vi "Main.vi"(11 "Module Admin":refnum<class "Delacor_lib_QMH_Module Admin.lvclass">) -> ()   [LabVIEW 2019, in "CONFIGURATION.lvlib"]
doc: "This template is based off of the Queued Message Handler design pattern and the Queued Message Handler project template that ships with LabVIEW.\n\nThe main difference is that the queue is private to this module and communication between modules is performed via Broadcast and Request events.\n\nRequest events are wrapped in public API methods and are handled in the Event Handling Loop (EHL) of this VI. Any module can register for Broadcast events sent by this module. The EHL generates messages based on user interface actions.\n\nThe Message Handling Loop (MHL) processes messages generated by the EHL, or by other messages. The messages are string values, so new messages can be added easily to the Message Cases case structure in the MHL. Each message cluster can also provide an optional value for Message Data, which is a variant that can be converted to whatever message-specific data is required.\n_____\nBased on Delacor QMH Project Template 5.0.0.82."
uses:
  CONFIGURATION.lvlib
  <vilib>/Delacor/Delacor QMH/Libraries/Module Admin_class/Delacor_lib_QMH_Module Admin.lvclass
  Module Data--cluster.ctl
  Stop Argument--cluster.ctl
  <vilib>/Delacor/Delacor QMH/Libraries/Message Queue_class/Delacor_lib_QMH_Message Queue.lvclass/Delacor_lib_QMH_Message Queue.ctl
  SET CONFIGURATIO Argument--cluster.ctl
  SAVE IN DB Argument--cluster.ctl
  DB_VENDING MACHINE/Type Defs/MONEY.ctl
  DB_VENDING MACHINE/Type Defs/PRODUCTS.ctl
  UPDATE DB TO MONEY LIST Argument--cluster.ctl
  SAVE PRODUCT IN DATABASE Argument--cluster.ctl
  UPDATE DB TO PRODUCT LIST Argument--cluster.ctl
  <vilib>/Utility/miscctls.llb/LVPointTypeDef.ctl
  <vilib>/Delacor/Delacor QMH/Libraries/Module Admin_class/Delacor_lib_QMH_Module Admin.lvclass/Delacor_lib_QMH_Module Admin.ctl
  <vilib>/Delacor/Delacor QMH/Libraries/Message Queue_class/Delacor_lib_QMH_Enqueue Message (Single).vi
  <vilib>/Delacor/Delacor QMH/Libraries/Module Admin_class/Delacor_lib_QMH_Get External Launch.vi
  <vilib>/Utility/error.llb/Error Cluster From Error Code.vi
  <vilib>/ErrorRing/Error Ring.xnode
  <vilib>/Delacor/Delacor QMH/Libraries/Message Queue_class/Delacor_lib_QMH_Message Queue.lvclass
  DB_VENDING MACHINE/DB_VENDING MACHINE.lvlib
  <vilib>/addons/database/NI_Database_API.lvlib
  COINS/COINS.lvlib
  MESSAGES/MESSAGES.lvlib
  Products/Products.lvlib
panel:
  in  "array 2":string[](array[string])
  in  "Tab Control":enum32{"MONEY", "PRODUCTS"}(tab)
  in  "SAVE MONEY IN DATABASE":bool
  in  "REMOVE COIN":bool
  in  "ADD COIN":bool
  in  "VALUE":dbl
  in  "DENOMINATION":string
  in  "Multicolumn MONEY":i32(listbox)
  in  "array":string[](array[string])
  out "MONEY":string[](array[string])
  in  "PRODUCTS":i32(listbox)
  in  "QUANTITY":i8
  in  "COST":dbl
  in  "PRODUCT":string
  in  "DELETE":bool
  in  "SAVE PRODUCT IN DATABASE":bool
  in  "SET CONFIG":bool
  out "error out":errorcluster
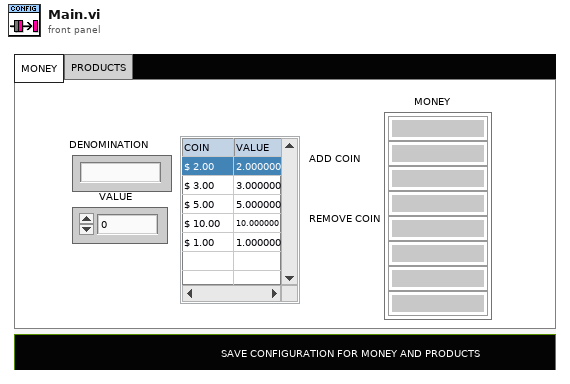
[diagram p1: front panel]
types:
  T1 = typedef "CONFIGURATION.lvlib/Request Events--cluster.ctl" = cluster{"Stop Module":refnum<user-event>, "Show Panel":refnum<user-event>, "Hide Panel":refnum<user-event>, "Get Module Execution Status":refnum<user-event>, "Show Diagram":refnum<user-event>, "SET CONFIGURATIO":refnum<user-event>, "UPDATE DB TO MONEY LIST":refnum<user-event>, "SAVE IN DB":refnum<user-event>, "SAVE PRODUCT IN DATABASE":refnum<user-event>, "UPDATE DB TO PRODUCT LIST":refnum<user-event>}
  T2 = typedef "CONFIGURATION.lvlib/Module Data--cluster.ctl" = cluster{"Status":string, "Money Array":string[]}
  T3 = enum32{"invalid lock state", "Not Locked", "Locked (No Password)", "Password-protected"}
  T4 = typedef "CONFIGURATION.lvlib/Stop Argument--cluster.ctl" = cluster{"Origin":string, "Exit via Stop Module Req?":bool, "Wait for Module to stop?":bool}
  T5 = typedef "CONFIGURATION.lvlib/SET CONFIGURATIO Argument--cluster.ctl" = cluster{"PRODUCTS":cluster{"PRODUCT":string, "COST":dbl, "QUANTITY":i8}, "MONEY":cluster{"COIN":string, "VALUE":dbl}, "MONEY ARRAY":string[]}
  T6 = typedef "DB_VENDING MACHINE.lvlib/MONEY.ctl" = cluster{"COIN":string, "MONEY":dbl}
  T7 = typedef "CONFIGURATION.lvlib/SAVE IN DB Argument--cluster.ctl" = cluster{"MONEY":T6, "PRODUCTS":T8, "DB?":bool}
  T8 = typedef "DB_VENDING MACHINE.lvlib/PRODUCTS.ctl" = cluster{"PRODUCT":string, "COST":dbl, "QUANTITY":i8}
  T9 = typedef "CONFIGURATION.lvlib/UPDATE DB TO MONEY LIST Argument--cluster.ctl" = cluster{"MONEY":T6}
  T10 = typedef "CONFIGURATION.lvlib/SAVE PRODUCT IN DATABASE Argument--cluster.ctl" = cluster{"PRODUCTS":T8}
  T11 = typedef "CONFIGURATION.lvlib/UPDATE DB TO PRODUCT LIST Argument--cluster.ctl" = cluster{"PRODUCTS":T8}
  T12 = enum32{"Invalid", "Standard", "Closed", "Hidden", "Minimized", "Maximized"}
  T13 = cluster{"PRODUCT":string, "COST":dbl, "QUANTITY":i8}
  T14 = typedef "LVPointTypeDef.ctl" = cluster{"Horizontal":i16, "Vertical":i16}
  T15 = typedef "NI_Database_API.lvlib/Conn ObjectReference.ctl" = refnum<k1>
  T16 = cluster{"array 2[0]":string, "array 2[1]":string, "array 2[2]":string, "array 2[3]":string, "array 2[4]":string, "array 2[5]":string, "array 2[6]":string, "array 2[7]":string, "array 2[8]":string}
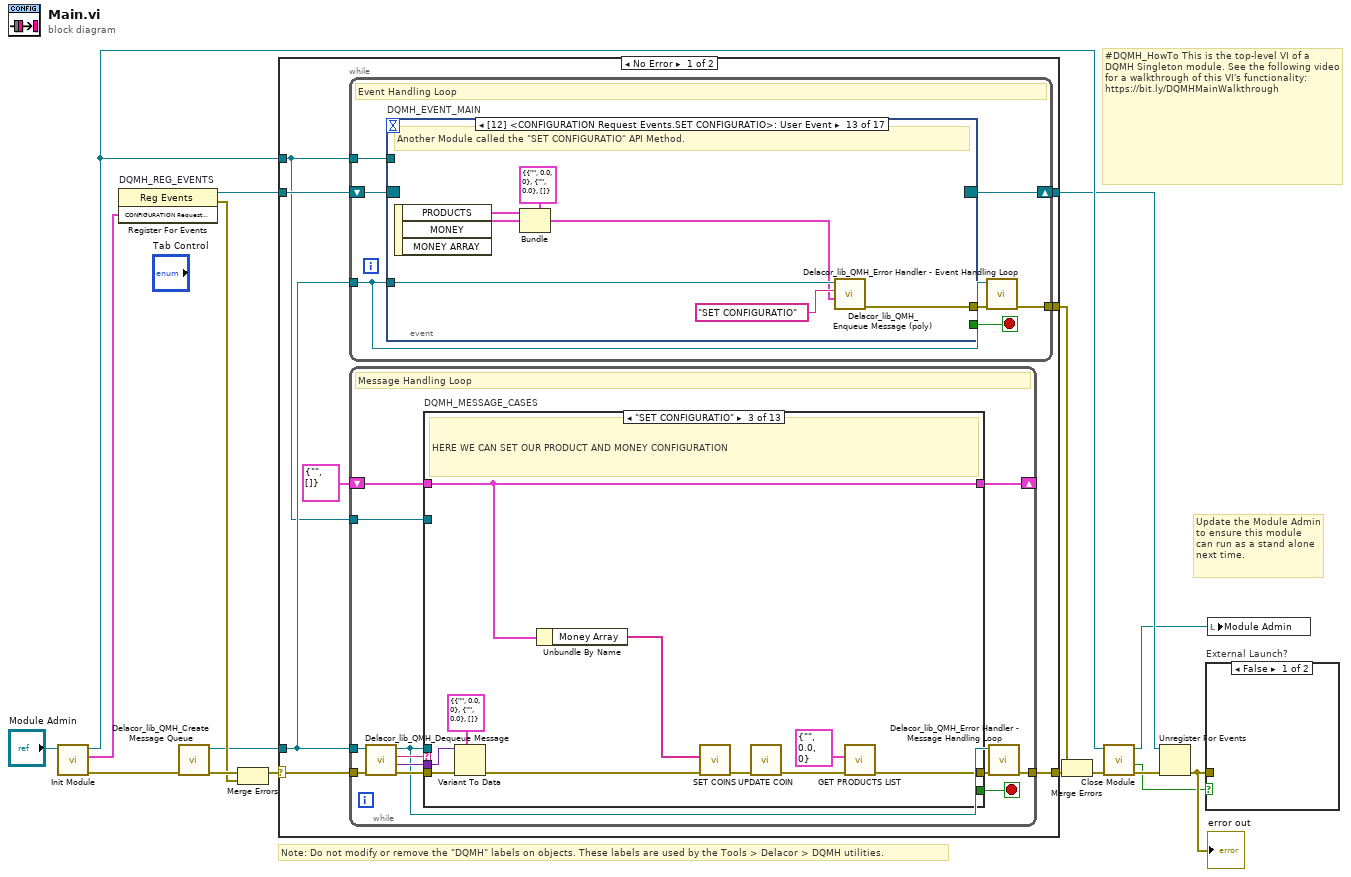
[diagram p0: block diagram]
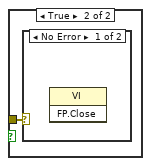
[diagram p2: hidden frame]
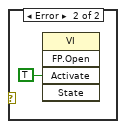
[diagram p3: hidden frame]
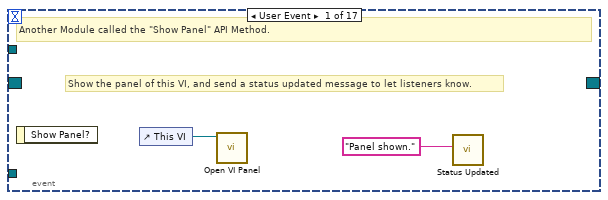
[diagram p4: hidden frame]
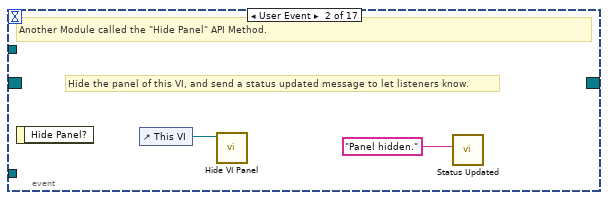
[diagram p5: hidden frame]
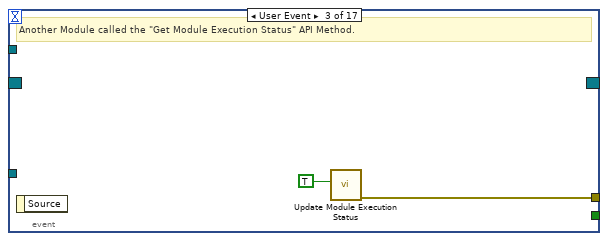
[diagram p6: hidden frame]
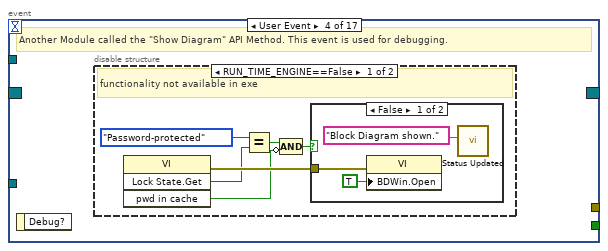
[diagram p7: hidden frame]
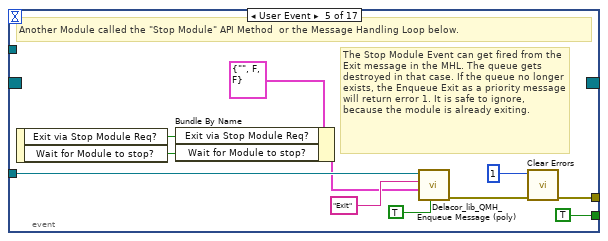
[diagram p10: hidden frame]
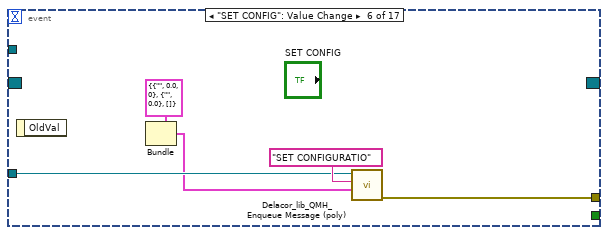
[diagram p11: hidden frame]
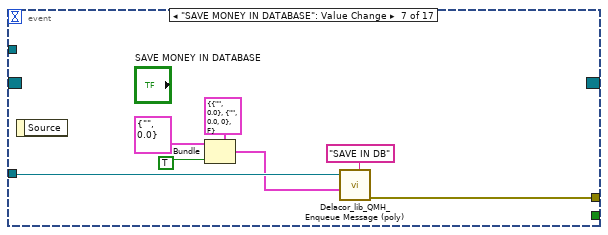
[diagram p12: hidden frame]
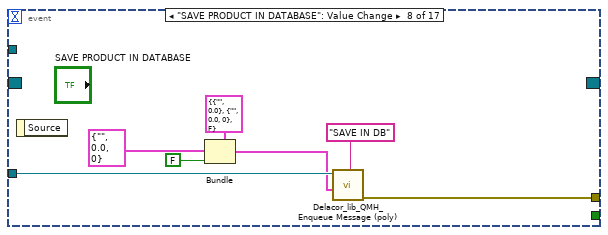
[diagram p13: hidden frame]
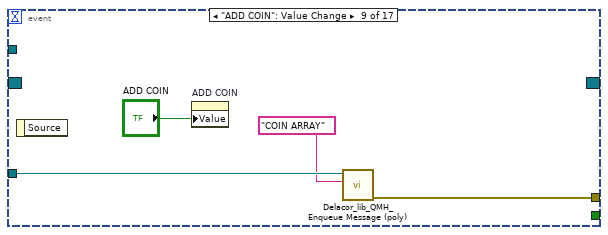
[diagram p14: hidden frame]
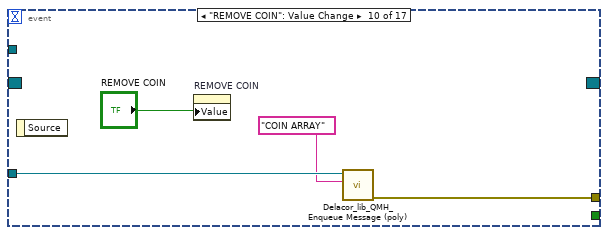
[diagram p15: hidden frame]
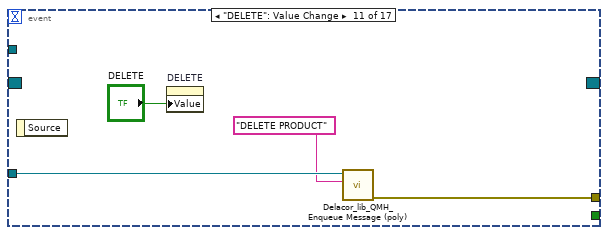
[diagram p16: hidden frame]
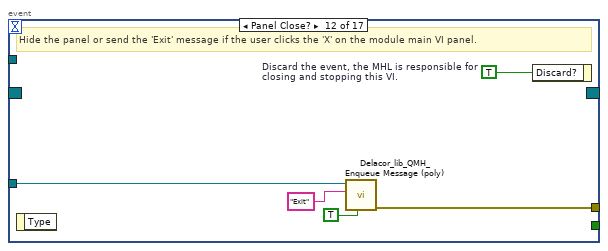
[diagram p17: hidden frame]
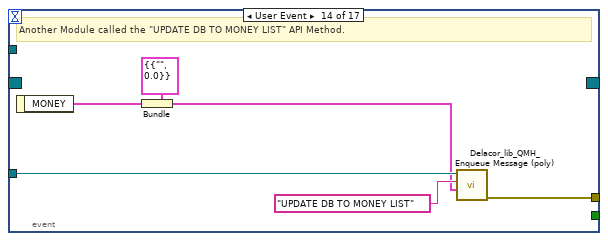
[diagram p18: hidden frame]
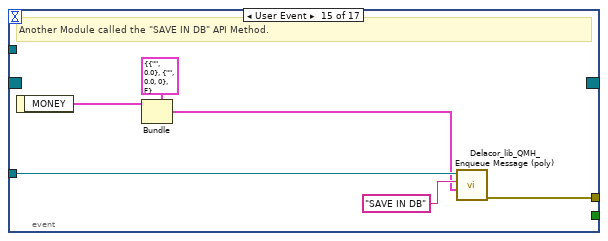
[diagram p19: hidden frame]
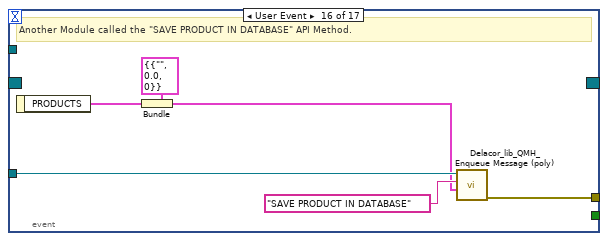
[diagram p20: hidden frame]
diagram:
  # "#DQMH_HowTo This is the top-level VI of a DQMH Singleton module. See the following video for a walkthrough of this VI's functionality: https://bit.ly/DQMHMainWalkthrough"
  # "Note: Do not modify or remove the \"DQMH\" labels on objects. These labels are used by the Tools > Delacor > DQMH utilities."
  # "Update the Module Admin to ensure this module can run as a stand alone next time."
  n1 = call "Init Module.vi"("Singleton Module Admin in"="Module Admin") -> ("error out"=w16:errorcluster, "CONFIGURATION Request Events"=w5:T1, "Singleton Module Admin out"=w8:refnum<class "Delacor_lib_QMH_Module Admin.lvclass">)  [unwired: 8 in]
  n2 = register-events "DQMH_REG_EVENTS"(w5) -> (reference out=w6:refnum<event-registration>, error out=w9:errorcluster)  [unwired: 2 in]
  n3 = call <vilib>:"Delacor_lib_QMH_Create Message Queue.vi"("error in (no error)"=w16) -> ("error out"=w11:errorcluster, "Message Queue"=w4:refnum<class "Delacor_lib_QMH_Message Queue.lvclass">)  [unwired: 9 in]
  n4 = Merge Errors(w11, w9) -> (w10:errorcluster)
  n5 = case shown="No Error" w10 {
    selector: w10 -> [w23 w320]
    tunnel: [w25 w319] -> w17
    tunnel: [w22 w325] -> w7
    tunnel: w6 -> [w20 w325]
    tunnel: w4 -> [w19 w318]
    tunnel: [w24 _] -> w14
    tunnel: w8 -> [w18 w321]
    frame No Error {
      n6 = while {
        tunnel: w19 -> [w26]
        shift-right: [w29] -> w22
        shift-left: w20 -> [w30]
        tunnel: [w31] -> w24
        tunnel: w18 -> [w27]
        stop <- w28 stop-if-true
        # "Event Handling Loop"
        n7 = event "DQMH_EVENT_MAIN" shown="[12] <CONFIGURATION Request Events.SET CONFIGURATIO>: User Event" {
          selector: w30 -> [_ _ _ _ _ _ _ _ _ _ _ _ _ _ _ _ _]
          dyn-events: [_ _ _ _ _ _ _ _ _ _ _ _ _ _ _ _ _] -> w29
          timeout: _ -> [_ _ _ _ _ _ _ _ _ _ _ _ _ _ _ _ _]
          tunnel: [_ _ _ _ TRUE ("Discard?") _ _ _ _ _ _ _ _ _ _ _ _] -> w28
          tunnel: w26 -> [_ _ _ _ w54 w62 w66 w72 w81 w85 w89 w92 w101 w107 w113 w119 w125]
          tunnel: [_ _ w38 _ w57 w61 w64 w73 w78 w82 w86 w94 w95 w102 w108 w114 w120] -> w32
          tunnel: w27 -> [_ _ _ _ _ _ _ _ _ _ _ _ _ _ _ _ _]
          event User Event {
            # "Show the panel of this VI, and send a status updated message to let listeners know."
            # "Another Module called the \"Show Panel\" API Method."
            n8 = event-data() -> ()  [unwired: 1 in, 1 out]
            n9 = control-ref of="This VI"() -> (w34:refnum<vi>)
            n10 = call "Open VI Panel.vi"("VI"=w34) -> ()  [unwired: 10 in, 1 out]
            n11 = call "Status Updated.vi"("Status"="Panel shown." ("format string")) -> ()  [unwired: 10 in, 1 out]
          }
          event User Event {
            # "Hide the panel of this VI, and send a status updated message to let listeners know."
            # "Another Module called the \"Hide Panel\" API Method."
            n12 = event-data() -> ()  [unwired: 1 in, 1 out]
            n13 = control-ref of="This VI"() -> (w36:refnum<vi>)
            n14 = call "Hide VI Panel.vi"("VI"=w36) -> ()  [unwired: 10 in, 1 out]
            n15 = call "Status Updated.vi"("Status"="Panel hidden." ("format string")) -> ()  [unwired: 10 in, 1 out]
          }
          event User Event {
            # "Another Module called the \"Get Module Execution Status\" API Method."
            n16 = event-data() -> ()  [unwired: 1 in, 1 out]
            n17 = call "Update Module Execution Status.vi"("Running?"=TRUE) -> ("error out"=w38:errorcluster)  [unwired: 10 in]
          }
          event User Event {
            # "Another Module called the \"Show Diagram\" API Method. This event is used for debugging."
            n18 = event-data() -> ()  [unwired: 1 in, 1 out]
            n19 = disable-structure shown="RUN_TIME_ENGINE==False" {
              frame condition #0 (active) {
                # "functionality not available in exe"
                n20 = invoke class="VI" method="Lock State.Get"() -> (error out=w44:errorcluster, "Get Lock State"=w43:T3, "pwd in cache"=w40:bool)  [unwired: 4 in, 1 out]
                n21 = Equal?(x=T3."Password-protected", y=w43) -> (x = y?=w41:bool)
                n22 = Compound Arithmetic op=AND(w41, invert w40) -> (w39:bool)
                n23 = case shown="False" w39 {
                  tunnel: w44 -> [w47 _]
                  frame False {
                    n24 = property class="VI"(error in=w47, "BDWin.Open"=TRUE ("Block Diagram Window:Open")) -> ()  [unwired: 1 in, 2 out]
                    n25 = call "Status Updated.vi"("Status"="Block Diagram shown." ("format string")) -> ()  [unwired: 10 in, 1 out]
                  }
                  frame True {
                    # "Password-protected VI, and the password is not in the cache. Do not show the diagram."
                  }
                }
              }
              frame condition #1 {
              }
            }
          }
          event User Event {
            # "The Stop Module Event can get fired from the Exit message in the MHL. The queue gets destroyed in that case. If the queue no longer exists, the Enqueue Exit as a priority message will return error 1. It is safe to ignore, because the module is already exiting."
            # "Another Module called the \"Stop Module\" API Method  or the Message Handling Loop below."
            n26 = event-data() -> ("Exit via Stop Module Req?"=w50:bool, "Wait for Module to stop?"=w49:bool)  [unwired: 1 in]
            n27 = Bundle By Name(cluster=T4 {"Origin"="", "Exit via Stop Module Req?"=FALSE, "Wait for Module to stop?"=FALSE} ("Stop Argument"), "Exit via Stop Module Req?"=w50, "Wait for Module to stop?"=w49) -> (w48:T4)
            n28 = call-poly <vilib>:"Delacor_lib_QMH_Enqueue Message (poly).vi"("Priority Message? (F)"=TRUE, "Message Data"=w48, "Message"="Exit", "Message Queue in"=w54) -> ("error out"=w58:errorcluster)  [unwired: 6 in, 1 out]
            n29 = call <vilib>:"Clear Errors.vi"("error in (no error)"=w58, "specific error code to clear (0: all)"=1) -> ("error out"=w57:errorcluster)  [unwired: 4 in, 1 out]
          }
          event "SET CONFIG": Value Change {
            n30 = event-data() -> ()  [unwired: 1 in, 1 out]
            n31 = Bundle(cluster=T5 {"PRODUCTS"={"PRODUCT"="", "COST"=0.0, "QUANTITY"=0}, "MONEY"={"COIN"="", "VALUE"=0.0}, "MONEY ARRAY"=[]} ("SET CONFIGURATIO Argument")) -> (w59:T5)  [unwired: 3 in]
            n32 = call-poly <vilib>:"Delacor_lib_QMH_Enqueue Message (poly).vi"("Message Data"=w59, "Message"="SET CONFIGURATIO", "Message Queue in"=w62) -> ("error out"=w61:errorcluster)  [unwired: 7 in, 1 out]
          }
          event "SAVE MONEY IN DATABASE": Value Change {
            n33 = event-data() -> ()  [unwired: 1 in, 1 out]
            n34 = Bundle(cluster=T7 {"MONEY"={"COIN"="", "MONEY"=0.0}, "PRODUCTS"={"PRODUCT"="", "COST"=0.0, "QUANTITY"=0}, "DB?"=FALSE} ("SAVE IN DB Argument"), "MONEY"=T6 {"COIN"="", "MONEY"=0.0}, "DB?"=TRUE) -> (w65:T7)  [unwired: 1 in]
            n35 = call-poly <vilib>:"Delacor_lib_QMH_Enqueue Message (poly).vi"("Message Data"=w65, "Message"="SAVE IN DB", "Message Queue in"=w66) -> ("error out"=w64:errorcluster)  [unwired: 7 in, 1 out]
          }
          event "SAVE PRODUCT IN DATABASE": Value Change {
            n36 = event-data() -> ()  [unwired: 1 in, 1 out]
            n37 = Bundle(cluster=T7 {"MONEY"={"COIN"="", "MONEY"=0.0}, "PRODUCTS"={"PRODUCT"="", "COST"=0.0, "QUANTITY"=0}, "DB?"=FALSE} ("SAVE IN DB Argument"), "PRODUCTS"=T8 {"PRODUCT"="", "COST"=0.0, "QUANTITY"=0}, "DB?"=FALSE) -> (w71:T7)  [unwired: 1 in]
            n38 = call-poly <vilib>:"Delacor_lib_QMH_Enqueue Message (poly).vi"("Message Data"=w71, "Message"="SAVE IN DB", "Message Queue in"=w72) -> ("error out"=w73:errorcluster)  [unwired: 7 in, 1 out]
          }
          event "ADD COIN": Value Change {
            n39 = event-data() -> ()  [unwired: 1 in, 1 out]
            n40 = property on="ADD COIN" class="Bool (strict)"("Value"="ADD COIN") -> ()  [unwired: 2 in, 2 out]
            n41 = call-poly <vilib>:"Delacor_lib_QMH_Enqueue Message (poly).vi"("Message"="COIN ARRAY", "Message Queue in"=w81) -> ("error out"=w78:errorcluster)  [unwired: 8 in, 1 out]
          }
          event "REMOVE COIN": Value Change {
            n42 = event-data() -> ()  [unwired: 1 in, 1 out]
            n43 = property on="REMOVE COIN" class="Bool (strict)"("Value"="REMOVE COIN") -> ()  [unwired: 2 in, 2 out]
            n44 = call-poly <vilib>:"Delacor_lib_QMH_Enqueue Message (poly).vi"("Message"="COIN ARRAY", "Message Queue in"=w85) -> ("error out"=w82:errorcluster)  [unwired: 8 in, 1 out]
          }
          event "DELETE": Value Change {
            n45 = event-data() -> ()  [unwired: 1 in, 1 out]
            n46 = property on="DELETE" class="Bool (strict)"("Value"="DELETE") -> ()  [unwired: 2 in, 2 out]
            n47 = call-poly <vilib>:"Delacor_lib_QMH_Enqueue Message (poly).vi"("Message"="DELETE PRODUCT", "Message Queue in"=w89) -> ("error out"=w86:errorcluster)  [unwired: 8 in, 1 out]
          }
          event Panel Close? {
            w93 = TRUE  # Discard the event, the MHL is responsible for closing and stopping this VI.
            # "Hide the panel or send the 'Exit' message if the user clicks the 'X' on the module main VI panel."
            n48 = event-data() -> ()  [unwired: 1 in, 1 out]
            n49 = call-poly <vilib>:"Delacor_lib_QMH_Enqueue Message (poly).vi"("Priority Message? (F)"=TRUE, "Message"="Exit", "Message Queue in"=w92) -> ("error out"=w94:errorcluster)  [unwired: 7 in, 1 out]
            n50 = event-data("Discard?"=w93) -> ()  [unwired: 1 in, 1 out]
          }
          event User Event {
            # "Another Module called the \"SET CONFIGURATIO\" API Method."
            n51 = event-data() -> ("PRODUCTS"=w97:T13, "MONEY"=w96:cluster{"COIN":string, "VALUE":dbl})  [unwired: 1 in, 1 out]
            n52 = Bundle(cluster=T5 {"PRODUCTS"={"PRODUCT"="", "COST"=0.0, "QUANTITY"=0}, "MONEY"={"COIN"="", "VALUE"=0.0}, "MONEY ARRAY"=[]} ("SET CONFIGURATIO Argument"), "PRODUCTS"=w97, "MONEY"=w96) -> (w98:T5)  [unwired: 1 in]
            n53 = call-poly <vilib>:"Delacor_lib_QMH_Enqueue Message (poly).vi"("Message Data"=w98, "Message"="SET CONFIGURATIO", "Message Queue in"=w101) -> ("error out"=w95:errorcluster)  [unwired: 7 in, 1 out]
          }
          event User Event {
            # "Another Module called the \"UPDATE DB TO MONEY LIST\" API Method."
            n54 = event-data() -> ("MONEY"=w103:T6)  [unwired: 1 in]
            n55 = Bundle(cluster=T9 {"MONEY"={"COIN"="", "MONEY"=0.0}} ("UPDATE DB TO MONEY LIST Argument"), "MONEY"=w103) -> (w104:T9)
            n56 = call-poly <vilib>:"Delacor_lib_QMH_Enqueue Message (poly).vi"("Message Data"=w104, "Message"="UPDATE DB TO MONEY LIST", "Message Queue in"=w107) -> ("error out"=w102:errorcluster)  [unwired: 7 in, 1 out]
          }
          event User Event {
            # "Another Module called the \"SAVE IN DB\" API Method."
            n57 = event-data() -> ("MONEY"=w109:T6)  [unwired: 1 in]
            n58 = Bundle(cluster=T7 {"MONEY"={"COIN"="", "MONEY"=0.0}, "PRODUCTS"={"PRODUCT"="", "COST"=0.0, "QUANTITY"=0}, "DB?"=FALSE} ("SAVE IN DB Argument"), "MONEY"=w109) -> (w110:T7)  [unwired: 2 in]
            n59 = call-poly <vilib>:"Delacor_lib_QMH_Enqueue Message (poly).vi"("Message Data"=w110, "Message"="SAVE IN DB", "Message Queue in"=w113) -> ("error out"=w108:errorcluster)  [unwired: 7 in, 1 out]
          }
          event User Event {
            # "Another Module called the \"SAVE PRODUCT IN DATABASE\" API Method."
            n60 = event-data() -> ("PRODUCTS"=w115:T8)  [unwired: 1 in]
            n61 = Bundle(cluster=T10 {"PRODUCTS"={"PRODUCT"="", "COST"=0.0, "QUANTITY"=0}} ("SAVE PRODUCT IN DATABASE Argument"), "PRODUCTS"=w115) -> (w116:T10)
            n62 = call-poly <vilib>:"Delacor_lib_QMH_Enqueue Message (poly).vi"("Message Data"=w116, "Message"="SAVE PRODUCT IN DATABASE", "Message Queue in"=w119) -> ("error out"=w114:errorcluster)  [unwired: 7 in, 1 out]
          }
          event User Event {
            # "Another Module called the \"UPDATE DB TO PRODUCT LIST\" API Method."
            n63 = event-data() -> ("PRODUCTS"=w121:T8)  [unwired: 1 in]
            n64 = Bundle(cluster=T11 {"PRODUCTS"={"PRODUCT"="", "COST"=0.0, "QUANTITY"=0}} ("UPDATE DB TO PRODUCT LIST Argument"), "PRODUCTS"=w121) -> (w122:T11)
            n65 = call-poly <vilib>:"Delacor_lib_QMH_Enqueue Message (poly).vi"("Message Data"=w122, "Message"="UPDATE DB TO PRODUCT LIST", "Message Queue in"=w125) -> ("error out"=w120:errorcluster)  [unwired: 7 in, 1 out]
          }
        }
        n66 = call-dynamic "Delacor_lib_QMH_Error Handler - Event Handling Loop.vi"("error in (no error)"=w32, "Message Queue in"=w26) -> ("dup error in"=w31:errorcluster)  [unwired: 8 in, 1 out]
      }
      n67 = while {
        tunnel: w19 -> [w128]
        shift-right: [w132] -> _
        shift-left: T2 {"Status"="", "Money Array"=[]} ("Data Cluster") -> [w133]
        tunnel: w23 -> [w136]
        tunnel: [w134] -> w25
        tunnel: w18 -> [w126]
        stop <- w131 stop-if-true
        # "Message Handling Loop"
        n68 = call-dynamic "Delacor_lib_QMH_Dequeue Message.vi"("error in (no error)"=w136, "Message Queue in"=w128) -> ("error out"=w135:errorcluster, "Message Data"=w129:variant, "Message"=w130:string, "Message Queue out"=w127:refnum<class "Delacor_lib_QMH_Message Queue.lvclass">)  [unwired: 6 in]
        n69 = case "DQMH_MESSAGE_CASES" shown="\"SET CONFIGURATIO\"" w130 {
          selector: w130 -> [_ _ _ _ _ _ _ _ _ _ _ _ w305]
          tunnel: w127 -> [_ _ _ _ _ _ _ _ _ _ w275 w297 _]
          tunnel: w135 -> [w157 w161 w171 w185 w197 w214 w242 w266 w269 w271 w282 w303 w307]
          tunnel: [w140 w161 w163 w174 w186 w214 w241 w255 w268 w271 w278 w300 w308] -> w137
          tunnel: w133 -> [w147 w160 w168 w184 w196 w217 w243 w253 w267 w270 w277 w296 w306]
          tunnel: [w147 w160 w168 w184 w196 w216 w243 w253 w267 w270 w277 w296 w306] -> w132
          tunnel: [_ _ _ _ _ _ _ _ _ _ _ w295 _] -> w131
          tunnel: w129 -> [_ _ w170 w182 w195 _ _ w264 _ _ w276 w294 _]
          tunnel: w126 -> [w148 _ _ _ _ _ _ _ _ _ w274 w289 _]
          frame "Initialize" {
            (unwired) T14 {"Horizontal"=0, "Vertical"=0} ("Origin")
            # "Initialize - Any operation that needs to be done before the module can receive messages. Synchronize Caller Events.vi will inform Start Module.vi that the module has launched and is ready to receive messages. Module Did Init.vi will broadcast that the module initialized."
            n70 = call "Synchronize Caller Events.vi"("error in (no error)"=w157, "Singleton Module Admin in"=w148) -> ("error out"=w156:errorcluster, "Singleton Module Admin out"=w144:refnum<class "Delacor_lib_QMH_Module Admin.lvclass">)  [unwired: 8 in]
            n71 = property class="Module Admin"(reference=w144) -> ("Accessors:External Launch"=w152:bool)  [unwired: 1 in, 2 out]
            n72 = Select(t=T12."Hidden" ("State"), s=w152, f=T12."Standard" ("State")) -> (s? t:f=w149:T12)
            n73 = call "Module Name--constant.vi"() -> ("Module Name"=w145:string)  [unwired: 11 in]
            n74 = call "SET MESSAGE.vi"("Message"="SETTING UP VENDING MACHINE") -> ()  [unwired: 10 in, 1 out]
            n75 = call "Module Name--constant.vi"() -> ("Module Name"=w155:string)  [unwired: 11 in]
            n76 = call "Module Did Init.vi"("error in (no error)"=w156, "Initialized?"=TRUE, "Origin"=w145) -> ("error out"=w143:errorcluster)  [unwired: 8 in]
            n77 = property class="VI"("Front Panel.Title"=w155) -> (reference out=w154:refnum<vi>, error out=w159:errorcluster)  [unwired: 2 in]
            n78 = invoke class="VI" method="FP.Open"(reference=w154, error in=w159, "State"=w149) -> (reference out=w153:refnum<vi>, error out=w158:errorcluster)  [unwired: 2 in, 3 out]
            n79 = call "UPDATE DB TO MONEY LIST.vi"("error in (no error)"=w143, "MONEY"=T6 {"COIN"="", "MONEY"=0.0}) -> ("error out"=w142:errorcluster)  [unwired: 9 in]
            n80 = invoke class="VI" method="FP.Center"(reference=w153, error in=w158) -> ()  [unwired: 1 in, 3 out]
            n81 = call "UPDATE DB TO PRODUCT LIST.vi"("error in (no error)"=w142, "PRODUCTS"=T8 {"PRODUCT"="", "COST"=0.0, "QUANTITY"=0}) -> ("error out"=w140:errorcluster)  [unwired: 9 in]
          }
          frame "--- Module Specific ---" {
            # "Separator -- The following cases handle messages specific to this Module."
          }
          frame "SET CONFIGURATIO" {
            # "HERE WE CAN SET OUR PRODUCT AND MONEY CONFIGURATION"
            n82 = Variant To Data(error in=w171, type=T5 {"PRODUCTS"={"PRODUCT"="", "COST"=0.0, "QUANTITY"=0}, "MONEY"={"COIN"="", "VALUE"=0.0}, "MONEY ARRAY"=[]} ("SET CONFIGURATIO Argument"), Variant=w170) -> (error out=w165:errorcluster)  [unwired: 1 out]
            n83 = Unbundle By Name(w168) -> ("Money Array"=w167:string[])
            n84 = call "SET COINS.vi"("error in (no error)"=w165, "MONEY ARRAY"=w167) -> ("error out"=w166:errorcluster)  [unwired: 8 in, 1 out]
            n85 = call "UPDATE COIN.vi"("error in (no error)"=w166) -> ("error out"=w164:errorcluster)  [unwired: 10 in]
            n86 = call "GET PRODUCTS LIST.vi"("error in (no error)"=w164, "PRODUCTS"=T8 {"PRODUCT"="", "COST"=0.0, "QUANTITY"=0}) -> ("error out"=w163:errorcluster)  [unwired: 9 in]
          }
          frame "UPDATE DB TO MONEY LIST" {
            # "HERE WE CAN UPDATE FROM DB OUR MONEY IN A LIST"
            n87 = Variant To Data(error in=w185, type=T9 {"MONEY"={"COIN"="", "MONEY"=0.0}} ("UPDATE DB TO MONEY LIST Argument"), Variant=w182) -> (data=w180:T9, error out=w183:errorcluster)
            n88 = Unbundle By Name(w180) -> ("MONEY"=w172:T6)
            n89 = control-ref of="Multicolumn MONEY"() -> (w179:refnum<vi>)
            n90 = call "DB_GET TABLE.vi"("MONEY"=w172) -> ("error out"=w177:errorcluster, "Array"=w178:string[][], "columns"=w175:string[], "Refnum out"=w176:T15)  [unwired: 7 in]
            n91 = call <vilib>:"DB Tools Close Connection.vi"("error in (no error)"=w177, "connection reference"=w176) -> ("error out"=w173:errorcluster)  [unwired: 5 in]
            n92 = Merge Errors(w173, w183) -> (w174:errorcluster)
            n93 = property class="MCListbox (strict)"(reference=w179, "ColHdrString"=w175, "ItemNames"=w178) -> ()  [unwired: 1 in, 2 out]
          }
          frame "SAVE IN DB" {
            # "HERE WE CAN SAVE NEW COINS AND VALUES"
            n94 = Variant To Data(error in=w197, type=T7 {"MONEY"={"COIN"="", "MONEY"=0.0}, "PRODUCTS"={"PRODUCT"="", "COST"=0.0, "QUANTITY"=0}, "DB?"=FALSE} ("SAVE IN DB Argument"), Variant=w195) -> (data=w190:T7, error out=w187:errorcluster)
            n95 = Unbundle By Name(w190) -> ("MONEY"=w192:T6, "PRODUCTS"=w191:T8, "DB?"=w188:bool)
            n96 = case shown="False" w188 {
              tunnel: [_ w210] -> w193
              tunnel: w192 -> [_ w209]
              tunnel: w191 -> [w205 _]
              tunnel: [w204 _] -> w189
              tunnel: w187 -> [w199 w207]
              tunnel: [w198 w206] -> w186
              frame False {
                n97 = Bundle By Name(cluster=w205, "PRODUCT"="PRODUCT", "COST"="COST", "QUANTITY"="QUANTITY") -> (w204:T8)
                n98 = call "UPDATE DB TO PRODUCT LIST.vi"("error in (no error)"=w199, "PRODUCTS"=T8 {"PRODUCT"="", "COST"=0.0, "QUANTITY"=0}) -> ("error out"=w198:errorcluster)  [unwired: 9 in]
              }
              frame True {
                n99 = Bundle By Name(cluster=w209, "COIN"="DENOMINATION", "MONEY"="VALUE") -> (w210:T6)
                n100 = call "UPDATE DB TO MONEY LIST.vi"("error in (no error)"=w207, "MONEY"=T6 {"COIN"="", "MONEY"=0.0}) -> ("error out"=w206:errorcluster)  [unwired: 9 in]
              }
            }
            n101 = call "DB_CONFIGURATION.vi"("TYPE ?"=w188, "PRODUCTS"=w189, "MONEY"=w193) -> ()  [unwired: 7 in, 2 out]
          }
          frame "COIN ARRAY" {
            n102 = property on="Multicolumn MONEY" class="MCListbox (strict)"() -> ("ItemNames"=w230:string[][])  [unwired: 2 in, 2 out]
            n103 = property on="ADD COIN" class="Bool (strict)"() -> ("Value"=w220:bool)  [unwired: 2 in, 2 out]
            n104 = Unbundle By Name(w217) -> ("Money Array"=w213:string[])
            "MONEY" <- w213
            n105 = property on="REMOVE COIN" class="Bool (strict)"() -> ("Value"=w221:bool)  [unwired: 2 in, 2 out]
            n106 = Index Array(array=w230, index (row)="Multicolumn MONEY") -> (element=w229:string[])  [unwired: 1 in]
            n107 = Select(t=1.0, s=w220, f=0.0) -> (s? t:f=w224:dbl)
            n108 = Select(t=-1.0, s=w221, f=0.0) -> (s? t:f=w223:dbl)
            n109 = Insert Into Array(array="array", new element=w229) -> (w219:string[])  [unwired: 1 in]
            n110 = Add(x=w224, y=w223) -> (x+y=w222:dbl)
            n111 = case shown="1" w222 {
              tunnel: w219 -> [_ w235 _]
              tunnel: [w232 w234 w236] -> w215
              tunnel: w213 -> [w232 w233 w237]
              frame 0, Default {
              }
              frame 1 {
                n112 = Insert Into Array(array=w233, new element=w235) -> (w234:string[])  [unwired: 1 in]
              }
              frame -1 {
                n113 = Delete From Array(array=w237, length=2) -> (array with subset deleted=w236:string[])  [unwired: 1 in, 1 out]
              }
            }
            n114 = Bundle By Name(cluster=w217, "Money Array"=w215) -> (w216:T2)
          }
          frame "DELETE PRODUCT" {
            n115 = property on="DELETE" class="Bool (strict)"() -> ("Value"=w239:bool)  [unwired: 2 in, 2 out]
            n116 = case shown="True" w239 {
              frame False {
              }
              frame True {
                n117 = property on="PRODUCTS" class="MCListbox (strict)"() -> ("ItemNames"=w251:string[][])  [unwired: 2 in, 2 out]
                n118 = Index Array(array=w251, index (row)="PRODUCTS") -> (element=w250:string[])  [unwired: 1 in]
                n119 = Insert Into Array(array="array 2", new element=w250) -> (w248:string[])  [unwired: 1 in]
                n120 = Array To Cluster(array=w248) -> (cluster=w247:T16)
                n121 = Unbundle By Name(w247) -> ("array 2[0]"=w246:string)
                n122 = Bundle By Name(cluster=T8 {"PRODUCT"="", "COST"=0.0, "QUANTITY"=0} ("PRODUCTS"), "PRODUCT"=w246) -> (w244:T8)
                n123 = call "DELETE_VENDING MACHINE.vi"("PRODUCTS"=w244) -> ()  [unwired: 10 in, 1 out]
              }
            }
            n124 = call "UPDATE DB TO PRODUCT LIST.vi"("error in (no error)"=w242, "PRODUCTS"=T8 {"PRODUCT"="", "COST"=0.0, "QUANTITY"=0}) -> ("error out"=w241:errorcluster)  [unwired: 9 in]
          }
          frame "UPDATE DB TO PRODUCT LIST" {
            # "HERE WE CAN SET DB DATA IN OUR PRODUCT LIST"
            n125 = Variant To Data(error in=w266, type=T11 {"PRODUCTS"={"PRODUCT"="", "COST"=0.0, "QUANTITY"=0}} ("UPDATE DB TO PRODUCT LIST Argument"), Variant=w264) -> (data=w262:T11, error out=w265:errorcluster)
            n126 = Unbundle By Name(w262) -> ("PRODUCTS"=w256:T8)
            n127 = control-ref of="PRODUCTS"() -> (w257:refnum<vi>)
            n128 = call "DB_GET PRODUCT TABLE.vi"("PRODUCTS"=w256) -> ("error out"=w260:errorcluster, "Array"=w261:string[][], "columns"=w258:string[], "Refnum out"=w259:T15)  [unwired: 7 in]
            n129 = call <vilib>:"DB Tools Close Connection.vi"("error in (no error)"=w260, "connection reference"=w259) -> ("error out"=w254:errorcluster)  [unwired: 5 in]
            n130 = property class="MCListbox (strict)"(reference=w257, "ColHdrString"=w258, "ItemNames"=w261) -> ()  [unwired: 1 in, 2 out]
            n131 = Merge Errors(w254, w265) -> (w255:errorcluster)
          }
          frame "---Copy This Frame---" {
            # "Duplicate this frame when creating new messages.  Change this comment in the duplicated frame to describe this message."
            n132 = Merge Errors(w269) -> (w268:errorcluster)
          }
          frame "--- Exit and Error Handling---" {
            # "Separator - The following cases handle errors and exit messages."
          }
          frame "Error" {
            # "#CodeRecommended - If you ever change the name of this \"Error\" message, you'll need to update the name in the Check Loop Error.vi as well."
            # "#CodeRecommended - If the module is running in standalone mode (External Launch = FALSE), this code will pop up an error dialog and call the 'Exit' message if an error occurs. Add more fine-grained error handling here."
            # "Error - Check the error message data and respond accordingly. This message is sent by the \"Error Handler\" VIs at the end of each loop in this application."
            n133 = property class="Module Admin"(reference=w274) -> ("Accessors:External Launch"=w273:bool)  [unwired: 1 in, 2 out]
            n134 = Variant To Data(error in=w282, type=errorcluster {"status"=FALSE, "code"=0, "source"=""} ("error constant"), Variant=w276) -> (data=w283:errorcluster, error out=w280:errorcluster)
            n135 = call "Module Name--constant.vi"() -> ("Module Name"=w272:string)  [unwired: 11 in]
            n136 = call "Error Reported.vi"("Additional Information"=w272, "Error"=w283) -> ()  [unwired: 9 in, 1 out]
            n137 = case shown="False" w273 {
              tunnel: [w288 _] -> w279
              tunnel: w275 -> [w286 _]
              tunnel: w283 -> [w287 _]
              frame False {
                # "If the module is running standalone, then pop up an error dialog and call the \"Exit\" message."
                n138 = call <vilib>:"Simple Error Handler.vi"("error in (no error)"=w287) -> ()  [unwired: 4 in, 5 out]
                n139 = call-poly <vilib>:"Delacor_lib_QMH_Enqueue Message (poly).vi"("Priority Message? (F)"=TRUE, "Message"="Exit", "Message Queue in"=w286) -> ("error out"=w288:errorcluster)  [unwired: 7 in, 1 out]
              }
              frame True {
                # "If the module was launched externally, calling the Error Reported broadcast VI is the only action performed by the \"Error\" message. The module's caller can then process the error appropriately."
              }
            }
            n140 = Merge Errors(w280, w279) -> (w278:errorcluster)
            n141 = local write "error out"(w278) -> ()
          }
          frame "Exit" {
            w293 = 91  # 91: not all Exit messages will have an argument
            w295 = TRUE  # Stop the VI
            # "Release the message queue reference"
            # "#CodeNeeded - Add any required cleanup code here"
            # "Exit - Exit the application."
            n142 = Variant To Data(error in=w303, type=T4 {"Origin"="", "Exit via Stop Module Req?"=FALSE, "Wait for Module to stop?"=FALSE} ("Stop Argument"), Variant=w294) -> (data=w291:T4, error out=w299:errorcluster)
            n143 = call <vilib>:"Clear Errors.vi"("error in (no error)"=w299, "specific error code to clear (0: all)"=w293) -> ("error out"=w302:errorcluster)  [unwired: 4 in, 1 out]
            n144 = control-ref of="This VI"() -> (w290:refnum<vi>)
            n145 = call-dynamic "Delacor_lib_QMH_Release Message Queue.vi"("error in (no error)"=w302, "Message Queue"=w297) -> ("error out"=w301:errorcluster)  [unwired: 9 in]
            n146 = call "Handle Exit.vi"("Stop Argument"=w291, "Admin in"=w289, "VI reference"=w290) -> ("error out"=w298:errorcluster)  [unwired: 7 in, 1 out]
            n147 = Merge Errors(w301, w298) -> (w300:errorcluster)
          }
          frame Default {
            # "'Default' case only runs if there is a message that isn't defined in any of the other cases.  Output a programming error."
            n148 = call "Module Name--constant.vi"() -> ("Module Name"=w304:string)  [unwired: 11 in]
            n149 = xnode "Error Ring"("parameter 0"=w305, "parameter 1"=w304) -> ("error out"=w309:errorcluster)
            n150 = Merge Errors(w307, w309) -> (w308:errorcluster)
          }
        }
        n151 = call-dynamic "Delacor_lib_QMH_Error Handler - Message Handling Loop.vi"("error in (no error)"=w137, "Message Queue in"=w127) -> ("dup error in"=w134:errorcluster)  [unwired: 8 in, 1 out]
      }
    }
    frame Error {
      # "Synchronize Caller Events.vi will inform Start Module.vi that the module has launched and will let the code calling Start Module.vi register for broadcasts and would permit the caller receive the broadcast that an error occurred at launch time."
      n152 = call-dynamic "Delacor_lib_QMH_Release Message Queue.vi"("error in (no error)"=w320, "Message Queue"=w318) -> ("error out"=w319:errorcluster)  [unwired: 9 in]
      n153 = call "Synchronize Caller Events.vi"("Singleton Module Admin in"=w321) -> ("error out"=w326:errorcluster)  [unwired: 9 in, 1 out]
      n154 = call "Module Name--constant.vi"() -> ("Module Name"=w324:string)  [unwired: 11 in]
      n155 = Format Into String(format string="An error occurred during initialization. %s is no longer running.", w324) -> (resulting string=w322:string)  [unwired: 2 in, 1 out]
      n156 = Merge Errors(w319, w326) -> (w327:errorcluster)
      n157 = call "Error Reported.vi"("Additional Information"=w322, "Error"=w327) -> ()  [unwired: 9 in, 1 out]
    }
  }
  n158 = Merge Errors(w14, w17) -> (w13:errorcluster)
  n159 = call "Close Module.vi"("error in (no error)"=w13, "Module Admin in"=w8) -> ("error out"=w15:errorcluster, "External Launch"=w1:bool, "Module Admin out"=w2:refnum<class "Delacor_lib_QMH_Module Admin.lvclass">)  [unwired: 7 in]
  n160 = Unregister For Events(event registration refnum=w7, error in=w15) -> (error out=w12:errorcluster)
  "error out" <- w12
  n161 = case "External Launch?" shown="False" w1 {
    tunnel: w12 -> [_ w328]
    frame False {
    }
    frame True {
      n162 = case shown="No Error" w328 {
        frame No Error {
          n163 = invoke class="VI" method="FP.Close"() -> ()  [unwired: 3 in, 3 out]
        }
        frame Error {
          n164 = invoke class="VI" method="FP.Open"("Activate"=TRUE ("Activate?")) -> ()  [unwired: 4 in, 5 out]
        }
      }
    }
  }
  n165 = local write "Module Admin"(w2) -> ()
